vi "RunTurnCalculator.vi"(0 "Total Angle (rad)":dbl, 2 "Calibrated positions of fiducials [mm]":dbl[][](array[numeric])=[[-658.867386146, 115.937184375, -18.342965965], [-563.38738772, 115.95451918, -18.342965965], [-563.369748267, 18.796520782, -18.342965965], [-658.849746693, 18.779185977, -18.342965965], [-560.867387761, 115.954976697, -18.342965965], [-465.387389335, 115.972311502, -18.342965965], [-465.369749882, 18.814313103, -18.342965965], [-560.849748308, 18.796978298, -18.342965965], [-462.867389377, 115.972769019, -18.342965965], [-367.38739095, 115.990103824, -18.342965965], [-367.369751497, 18.832105425, -18.342965965], [-462.849749923, 18.81477062, -18.342965965], [-364.867390992, 115.990561341, -18.342965965], [-269.387392565, 116.007896146, -18.342965965], [-269.369753112, 18.849897747, -18.342965965], [-364.849751539, 18.832562942, -18.342965965], [-266.867392607, 116.008353663, -18.342965965], [-171.38739418, 116.025688468, -18.342965965], [-171.369754727, 18.867690069, -18.342965965], [-266.849753154, 18.850355264, -18.342965965], [-168.867394222, 116.026145985, -18.342965965], [-73.387395796, 116.04348079, -18.342965965], [-73.369756342, 18.885482391, -18.342965965], [-168.849754769, 18.868147586, -18.342965965], [-70.867395837, 116.043938306, -18.342965965], [24.612602589, 116.061273111, -18.342965965], [24.630242042, 18.903274713, -18.342965965], [-70.849756384, 18.885939908, -18.342965965], [27.132602548, 116.061730628, -18.342965965], [122.612600974, 116.079065433, -18.342965965], [122.630240427, 18.921067035, -18.342965965], [27.150242001, 18.90373223, -18.342965965], [125.132600933, 116.07952295, -18.342965965], [220.612599359, 116.096857755, -18.342965965], [220.630238812, 18.938859356, -18.342965965], [125.150240386, 18.921524551, -18.342965965], [223.132599318, 116.097315272, -18.342965965], [318.612597744, 116.114650077, -18.342965965], [318.630237197, 18.956651678, -18.342965965], [223.150238771, 18.939316873, -18.342965965], [321.132597702, 116.115107594, -18.342965965], [416.612596129, 116.132442399, -18.342965965], [416.630235582, 18.974444, -18.342965965], [321.150237156, 18.957109195, -18.342965965], [419.132596087, 116.132899916, -18.342965965], [514.612594514, 116.150234721, -18.342965965], [514.630233967, 18.992236322, -18.342965965], [419.15023554, 18.974901517, -18.342965965], [517.132594472, 116.150692238, -18.342965965], [612.612592899, 116.168027043, -18.342965965], [612.630232352, 19.010028644, -18.342965965], [517.150233925, 18.992693839, -18.342965965]], 3 "Corner surveyed position":dbl[](array[numeric]), 4 "Loading Tool":u16(ring) items=["Metric", "English"], 5 "Module number":i32) -> (1 "Update Led":bool=TRUE, 6 "Angle Knob Rotations":dbl, 7 "X Knob Rotations":dbl, 8 "Y Knob Rotations":dbl)   [LabVIEW 2017]
panel:
  out "Y side length":dbl
  out "X side length":dbl
  out "Corner D ideal":dbl[](array[numeric])
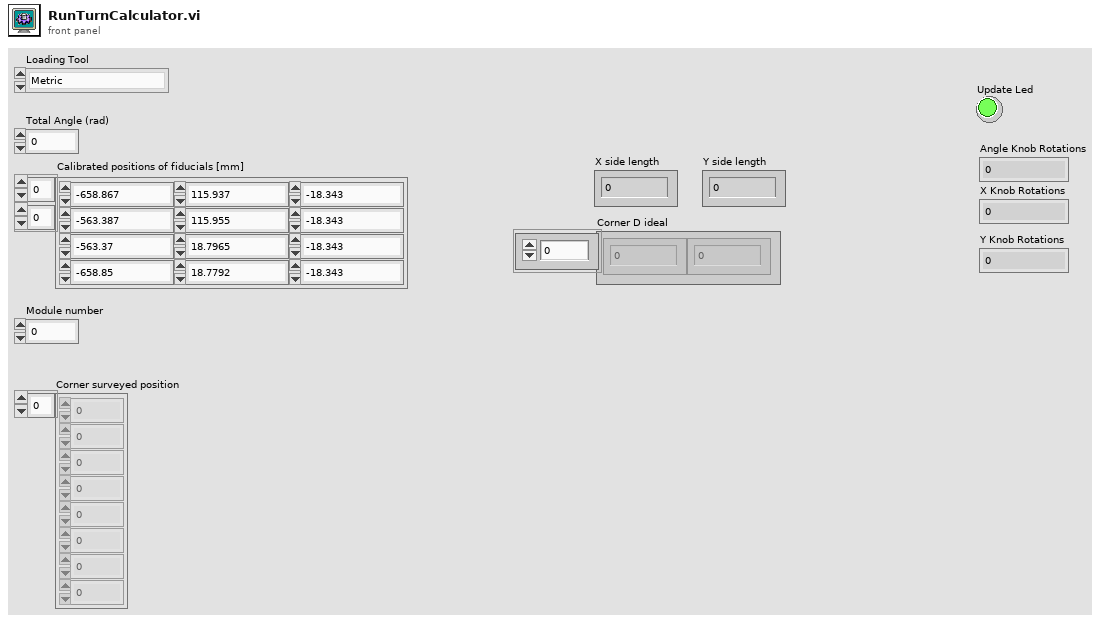
[diagram p1: front panel]
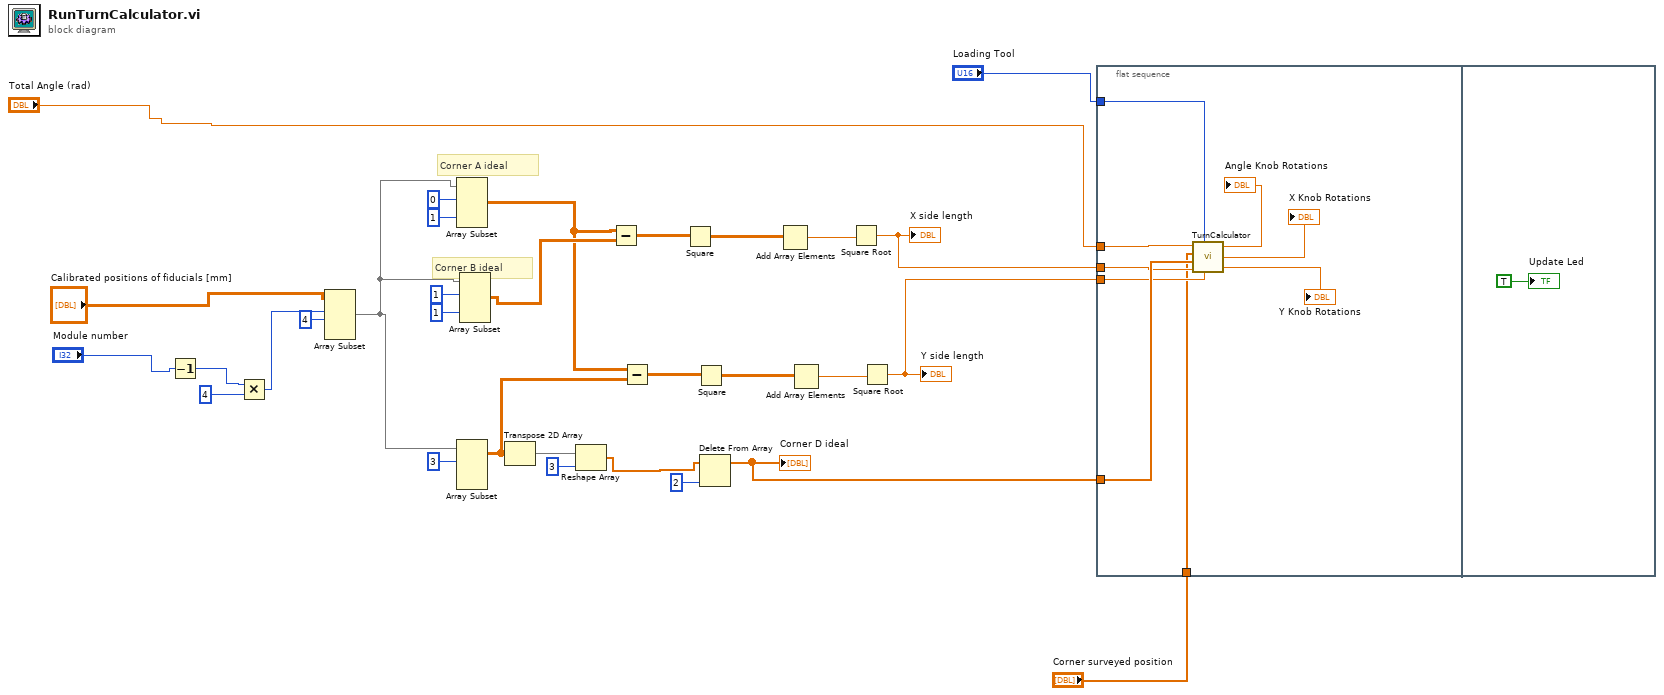
[diagram p0: block diagram]
diagram:
  # "Corner B ideal"
  # "Corner A ideal"
  n1 = Decrement(x="Module number") -> (x-1=w29:i32)
  n2 = Multiply(x=w29, y=4) -> (x*y=w27:i32)
  n3 = Array Subset(array="Calibrated positions of fiducials [mm]", index (row)=w27, length (row)=4 ("length")) -> (w18:dbl[][])  [unwired: 2 in]
  n4 = Array Subset(array=w18, index (row)=0 ("index"), length (row)=1 ("length")) -> (w8:dbl[][])  [unwired: 2 in]
  n5 = Array Subset(array=w18, index (row)=3 ("index")) -> (w7:dbl[][])  [unwired: 3 in]
  n6 = Array Subset(array=w18, index (row)=1 ("index"), length (row)=1 ("length")) -> (w17:dbl[][])  [unwired: 2 in]
  n7 = Transpose 2D Array(2D array=w7) -> (transposed array=w23:dbl[][])
  n8 = Reshape Array(w23, 3 ("dimension size")) -> (w22:dbl[])
  n9 = Subtract(x=w8, y=w17) -> (x-y=w16:dbl[][])
  n10 = Subtract(x=w8, y=w7) -> (x-y=w11:dbl[][])
  n11 = Square(x=w16) -> (x^2=w15:dbl[][])
  n12 = Square(x=w11) -> (x^2=w10:dbl[][])
  n13 = Delete From Array(array=w22, index=2) -> (array with subset deleted=w6:dbl[])  [unwired: 1 in, 1 out]
  "Corner D ideal" <- w6
  n14 = Add Array Elements(numeric array=w15) -> (sum=w14:dbl)
  n15 = Add Array Elements(numeric array=w10) -> (sum=w9:dbl)
  n16 = Square Root(x=w14) -> (sqrt(x)=w5:dbl)
  "X side length" <- w5
  n17 = Square Root(x=w9) -> (sqrt(x)=w4:dbl)
  "Y side length" <- w4
  n18 = flat-sequence {
    tunnel: w6 -> [w40]
    tunnel: w5 -> [w39]
    tunnel: w4 -> [w38]
    tunnel: "Corner surveyed position" -> [w34]
    tunnel: "Total Angle (rad)" -> [w33]
    tunnel: "Loading Tool" -> [w32]
    frame #0 {
      n19 = call "TurnCalculator.vi"("Desired Angle"=w33, "Loading Tool"=w32, "Measured Coordinates (mm)"=w34, "Top Left Corner Desired Coordinates (mm)"=w40, "Y Side length (m)"=w38, "X Side length (m)"=w39) -> ("Angle Knob Rotations"=→"Angle Knob Rotations":dbl, "X Knob Rotations"=→"X Knob Rotations":dbl, "Y Knob Rotations"=→"Y Knob Rotations":dbl)
    }
    frame #1 {
      "Update Led" <- TRUE
    }
  }
